vi "Get Out_Data.vi"(8 "error in (no error)":errorcluster caption="entrée d'erreur (pas d'erreur)", 11 "Firebase Packaging en entrée":refnum<class "Firebase Find_Batch_Fct_SN.lvclass">) -> (0 "error out":errorcluster caption="sortie d'erreur", 2 "Out_Data":T1, 3 "Firebase Packaging en sortie":refnum<class "Firebase Find_Batch_Fct_SN.lvclass">)   [LabVIEW 2020, in "Library Instrument & Equipement.lvlib" / "Library FireBase.lvlib" / "Firebase Find_Batch_Fct_SN.lvclass"]
uses:
  Firebase Find_Batch_Fct_SN.lvclass
  Firebase Find_Batch_Fct_SN.lvclass/Firebase Find_Batch_Fct_SN.ctl
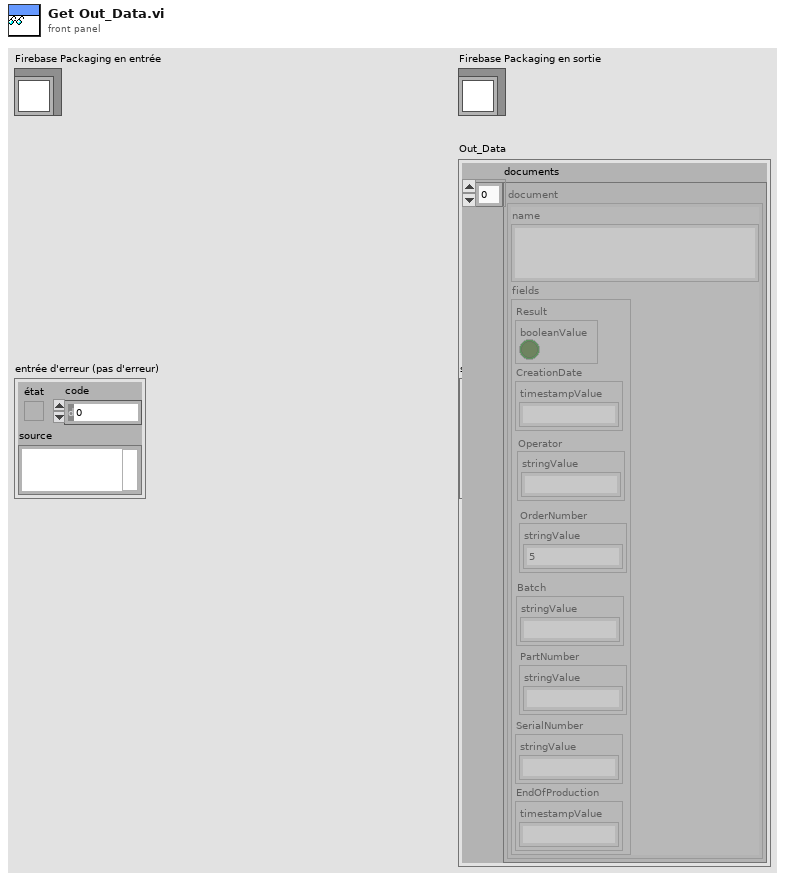
[diagram p1: front panel]
types:
  T1 = cluster{"documents":cluster{"name":string, "fields":cluster{"Result":cluster{"booleanValue":bool}, "CreationDate":cluster{"timestampValue":string}, "Batch":cluster{"stringValue":string}, "SerialNumber":cluster{"stringValue":string}, "EndOfProduction":cluster{"timestampValue":string}, "PartNumber":cluster{"stringValue":string}, "OrderNumber":cluster{"stringValue":string}, "Operator":cluster{"stringValue":string}}}[]}
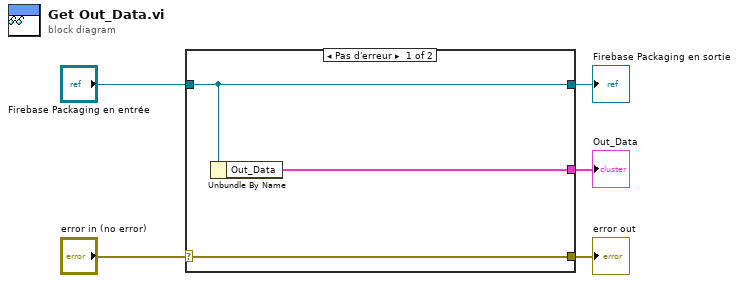
[diagram p0: block diagram]
diagram:
  n1 = case shown="Pas d'erreur" "error in (no error)" {
    selector: "error in (no error)" -> [w8 w9]
    tunnel: [w8 w9] -> w4
    tunnel: [w7 w10] -> w2
    tunnel: "Firebase Packaging en entrée" -> [w7 w10]
    tunnel: [w6 _] -> w1
    frame No Error {
      n2 = Unbundle By Name(w7) -> ("Out_Data"=w6:T1)
    }
    frame Error {
    }
  }
  "error out" <- w4
  "Firebase Packaging en sortie" <- w2
  "Out_Data" <- w1
